vi "exitControl.vi"(8 "error in (no error)":errorcluster, 10 "Model in":refnum<class "Model.lvclass">, 11 "StandbyState in":refnum<class "StandbyState.lvclass">) -> (0 "error out":errorcluster, 2 "Model out":refnum<class "Model.lvclass">, 3 "StandbyState out":refnum<class "StandbyState.lvclass">)   [LabVIEW 2016, in "StandbyState.lvclass"]
uses:
  StandbyState.lvclass
  Model/Model.lvclass
  Types/DetailedStates.ctl
  Types/M1M3SupportTypes.lvlib
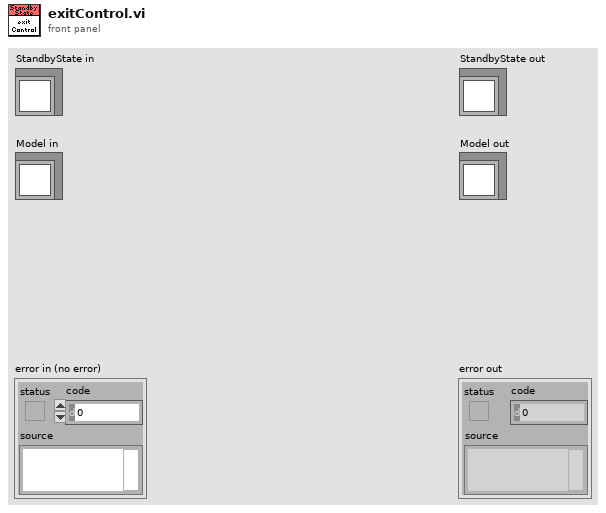
[diagram p1: front panel]
types:
  T1 = typedef "M1M3SupportTypes.lvlib/DetailedStates.ctl" = enum16{"PublishOnlyState", "AvailableState", "StandbyState", "DisabledState", "EnabledState", "FaultState"}
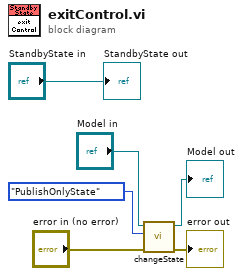
[diagram p0: block diagram]
diagram:
  n1 = call "changeState.vi"("error in (no error)"="error in (no error)", "DetailedStates"=DetailedStates."PublishOnlyState", "Model in"="Model in") -> ("error out"=→"error out":errorcluster, "Model out"=→"Model out":refnum<class "Model.lvclass">)  [unwired: 7 in]
  "StandbyState out" <- "StandbyState in"
